vi "Save_local_database.vi"(3 "error in (no error)":errorcluster, 5 "Data to add":T1) -> (0 "error out":errorcluster)   [LabVIEW 2019]
uses:
  <vilib>/addons/database/Connection.llb/DB Tools Open Connec (Path).vi
  Type defs/Database_control.ctl
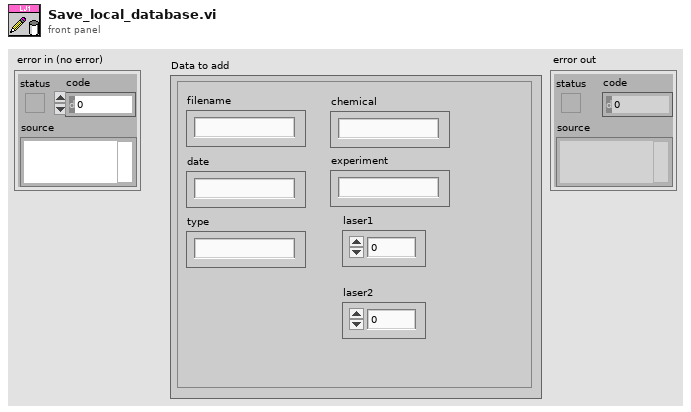
[diagram p1: front panel]
types:
  T1 = typedef "Database_control.ctl" = cluster{"filename":string, "date":string, "type":string, "chemical":string, "experiment":string, "laser1":dbl, "laser2":dbl}
  T2 = typedef "NI_Database_API.lvlib/Conn ObjectReference.ctl" = refnum<k1>
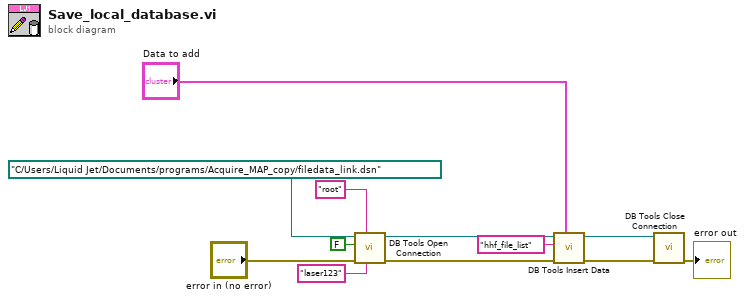
[diagram p0: block diagram]
diagram:
  n1 = call-poly <vilib>:"DB Tools Open Connection.vi"("password"="laser123", "userID"="root", "error in (no error)"="error in (no error)", "prompt? (F)"=FALSE, "connection information"=path "C:/Users/Liquid Jet/Documents/programs/Acquire_MAP_copy/filedata_link.dsn") -> ("error out"=w7:errorcluster, "connection reference"=w9:T2)  [unwired: 3 in]
  n2 = call <vilib>:"DB Tools Insert Data.vi"("data"="Data to add", "error in (no error)"=w7, "table"="hhf_file_list", "connection reference"=w9) -> ("error out"=w6:errorcluster, "connection reference out"=w8:T2)  [unwired: 6 in]
  n3 = call <vilib>:"DB Tools Close Connection.vi"("error in (no error)"=w6, "connection reference"=w8) -> ("error out"=→"error out":errorcluster)  [unwired: 5 in]
